vi "L1 Command Conversions.vi"(8 "error in (no error)":errorcluster, 10 "Inputs":dbl[](array[numeric]), 11 "ConversionOps":T1) -> (0 "error out":errorcluster, 2 "Outputs":dbl[](array[numeric]))   [LabVIEW 2013]
uses:
  Conversion Operations.ctl
  Data Access Objects/Metadata/DAO Actions with Remove.ctl
  Data Access Objects/Metadata/LBCB Number.ctl
  LbcbConversionTypes.ctl
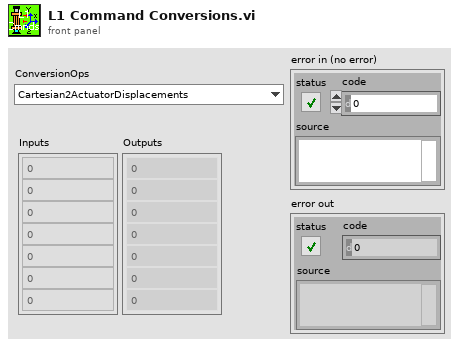
[diagram p1: front panel]
types:
  T1 = typedef "Conversion Operations.ctl" = enum16{"Cartesian2ActuatorDisplacements", "Actuator2CartesianDisplacements", "Actuators2CartesianForces", "Initialize"}
  T2 = typedef "LbcbConversionTypes.ctl" = enum16{"Commands", "Readings", "Offsets"}
  T3 = typedef "LBCB Number.ctl" = enum16{"LBCB1", "LBCB2"}
  T4 = typedef "DAO Actions with Remove.ctl" = enum16{"Init", "Get", "Set", "Remove"}
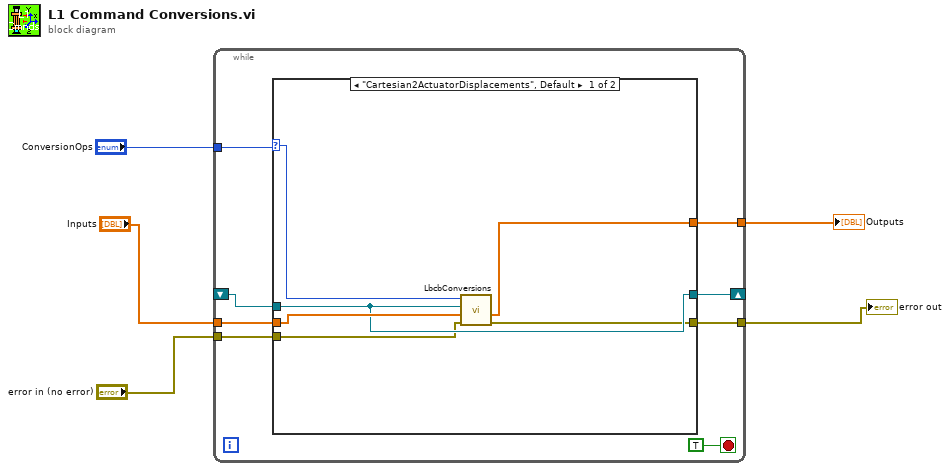
[diagram p0: block diagram]
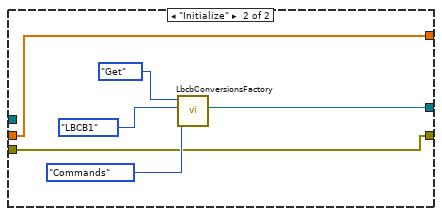
[diagram p2: hidden frame]
diagram:
  n1 = while {
    tunnel: "ConversionOps" -> [w12]
    shift-right: [w11] -> _
    shift-left: _ -> [w10]
    tunnel: "Inputs" -> [w9]
    tunnel: [w8] -> w3
    tunnel: [w7] -> w2
    tunnel: "error in (no error)" -> [w6]
    stop <- TRUE stop-if-true
    n2 = case shown="\"Cartesian2ActuatorDisplacements\", Default" w12 {
      selector: w12 -> [w19 _]
      tunnel: [w16 w25] -> w11
      tunnel: w10 -> [w16 _]
      tunnel: w9 -> [w18 w21]
      tunnel: [w17 w21] -> w8
      tunnel: [w15 w20] -> w7
      tunnel: w6 -> [w14 w20]
      frame "Cartesian2ActuatorDisplacements", Default {
        n3 = call "LbcbConversions.vi"("error in (no error)"=w14, "Inputs"=w18, "Conversion Ref"=w16, "ConversionOps"=w19) -> ("error out"=w15:errorcluster, "Outputs"=w17:dbl[])  [unwired: 6 in]
      }
      frame "Initialize" {
        n4 = call "LbcbConversionsFactory.vi"("LbcbConversionType"=LbcbConversionTypes."Commands", "LBCB Number"=LBCB_Number."LBCB1", "Actions"=DAO_Actions_with_Remove."Get") -> ("Conversion Ref"=w25:refnum<k24>)  [unwired: 7 in, 1 out]
      }
    }
  }
  "Outputs" <- w3
  "error out" <- w2
